vi "Main Tclk.vi"() -> ()   [LabVIEW 2018] (continued)
  T17 = cluster{"Filament (A)":sgl, "Accelerator Target (V)":sgl, "Accelerator Actual (V)":sgl, "Extrator Target (V)":sgl, "Extrator Actual (V)":sgl, "Emission Target (uA)":sgl, "Emission Actual (uA)":sgl, "Suppressor (V)":sgl, "Faraday I (nA)":sgl, "Lens1 Target (V)":sgl, "Lens1 Actual (V)":sgl, "Lens2 Target (V)":sgl, "Lens2 Actual (V)":sgl, "Gun Vac (Torr)":sgl, "Column Vac (Torr)":sgl, "Tip Lifetime (uAhr)":sgl}
  T18 = cluster{"Filament (A)":sgl, "Accelerator (V)":sgl, "AccI (uA)":sgl, "Extrator (V)":sgl, "Emission (uA)":sgl, "Suppressor (V)":sgl, "SuppI (uA)":sgl, "Lens1 (V)":sgl, "Lens1I (uA)":sgl, "Lens2 (V)":sgl, "Lens2I (uA)":sgl, "Tip Lifetime (hr)":sgl}
  T19 = cluster{"FIB mode":u8, "FIB focus":sgl, "FIB probe current":sgl, "FIB emission (uA)":sgl, "FIB rotation":sgl, "FIB aperture X":sgl, "FIB aperture Y":sgl, "FIB stig X":sgl, "FIB stig Y":sgl, "FIB beam shift X":sgl, "FIB beam shift Y":sgl}
  T20 = cluster{"Actual scan rate":dbl, "X resolution with rampdown":i32, "Actual sample rate":dbl, "Fetch backlog":dbl, "Total scan points":i32, "Frame rate (/s)":u32}
  T21 = cluster{"Reheat finish time":string, "Reheat Success":bool, "Initial emission (uA)":sgl, "Initial suppressor (V)":sgl, "V/I Slope":sgl}
  T22 = typedef "LVPoint32TypeDef.ctl" = cluster{"Horizontal":i32, "Vertical":i32}
  T23 = cluster{"FIB X coil":tag, "FIB Y coil":tag, "Beam blank":tag, "FIB Ext Scan":tag, "Detector":tag, "Shutter Drive":tag}
  T24 = enum32{"Hardware", "SEM", "Add'l SEM's", "File & Logging", "FIB Imaging", "FIB Reheat", "FIB Milling", "Alert"}
  T25 = cluster{"SEM X coil":refnum<k15>, "SEM Y coil":refnum<k15>, "FIB X coil":tag, "FIB Y coil":tag, "FIB Detector":tag, "SEM Detectors":refnum<k15>, "Det min (V)":dbl, "Det max (V)":dbl, "Eanable COM":bool, "COM port":refnum<visa-resource-name>, "FIB Beam blank":tag, "FIB Ext Scan":tag, "Det. FIB-NI auto switch":tag, "Shutter Drive":tag, "Machine Type":u8, "FIB Faraday Cup":tag, "Configuration file":path, "SEM Max FOV (um)":sgl, "Machine ID":string, "Save config file":bool, "Temperature port":refnum<visa-resource-name>, "Brightness A":dbl, "Contrast A":dbl, "Detector B name":string, "Brightness B":dbl, "Contrast B":dbl, "Logging Device":tag}
  T26 = cluster{"X size (um)":sgl, "Y size (um)":sgl, "X center (um)":sgl, "Y center (um)":sgl, "X size (V)":dbl, "X size auto":bool, "X stig":sgl[][], "Y stig":sgl[][], "X aln":sgl[][], "Y aln":sgl[][], "Scan rate (Hz)":u32, "Oversampling":u32, "Oversampling auto":bool, "Frame line rampdown ratio":sgl, "Pixel size (nm)":sgl, "WD (mm)":sgl[][], "X tiles":u8, "Y tiles":u8, "Overlap (um)":sgl, "Interlaced":bool, "dX (um)":sgl[], "dY (um)":sgl[], "Frames":u8}
  T27 = cluster{"GetInfo":bool, "Set Det A para":bool, "Set WD":bool, "Set Mag":bool, "Set stig":bool, "Set aln":bool, "Display":bool, "Save":bool, "8-bit":bool, "Detector A":bool, "Detector B":bool, "Detector C":bool, "Detector D":bool, "Inverse A":bool, "Inverse B":bool, "Inverse C":bool, "Inverse D":bool, "Inverse PNG":bool, "Freeze":bool, "PNG only":bool, "Upload":bool, "Delete after upload":bool}
  T28 = cluster{"Keep aspect ratio":bool, "Show Focus Index":bool, "Focus Index primary grid center":bool, "X Grids":u8[][], "Y Grids":u8[][], "Primary X index":u8[][], "Primary Y index":u8[][]}
  T29 = cluster{"Mid mag scan":bool, "Prior to main scan":bool, "Mid mag interval":u32, "X size (um)":sgl, "Y size (um)":sgl, "X center (um)":dbl, "Y center (um)":dbl, "Mid mag scan rate (Hz)":u32, "Pixel size (nm)":sgl, "Show MM box":bool}
  T30 = cluster{"Low mag scan":bool, "Prior to main scan":bool, "Low mag interval":u32, "Low mag scan FOV (micron)":dbl, "Low mag scan rate (Hz)":u32, "Show HM box":bool}
  T31 = cluster{"File path":path, "Notes":string, "Save recipe":bool, "Load recipe":bool, "Sample ID":string}
  T32 = cluster{"X resolution":u32, "Z resolution":u32, "X center":dbl, "Z center":dbl, "X size (V)":dbl, "Z size (V)":dbl, "Frame line rampdown ratio":dbl, "Scan rate (Hz)":u32, "Oversampling":u16}
  T33 = cluster{"Scan mode":u16, "Flip x":bool, "Flip z":bool, "Det":u16}
  T34 = cluster{"X resolution":u32, "Y resolution":u32, "X center":dbl, "Y center":dbl, "X size (V)":dbl, "Y size (V)":dbl, "Frame line rampdown ratio":dbl, "Scan rate (Hz)":u32, "Oversampling":u16}
  T35 = cluster{"X resolution":u32, "Z resolution":u32, "X offset (um)":sgl, "Z offset (um)":sgl, "X center (um)":sgl, "Z center (um)":sgl, "X size (um)":sgl, "Z size (um)":sgl, "UL-Ang":sgl, "UR-Ang":sgl, "Line milling time (s)":sgl, "Z-step (nm)":dbl, "Lines auto pause":u16, "Auto pause":bool, "Mill from Bottom":bool, "FIB FOV (um)":sgl, "Auto Profile":bool, "Mill start from Last":bool, "FIB PID on":bool, "FIB PID reset":bool, "FIB PID measured":u8, "FIB PID target":sgl, "FIB PID target slope":sgl, "FIB PID P":sgl, "FIB PID I":sgl, "FIB PID D":sgl, "Emission (uA)":dbl, "Suppressor (V)":sgl, "Auto reheat":bool}
  T36 = cluster{"3D imaging paused alarm":bool, "FIB emission warning":bool, "Low limit":dbl, "High limit":dbl, "Specimen @ SEM alarm":bool, "FIB CL current alarm":bool, "Beam Dump 1 alarm":bool, "Milling Z voltage alarm":bool, "EHT off alarm":bool, "Detector over scale warning":bool, "Image clipping alarm":bool, "Warning limit (um)":sgl, "Stop limit (um)":sgl, "Temperature alarm":bool, "Pause 3D-ING":bool, "Low limit (F)":sgl, "High limit (F)":sgl, "Temp limit auto":bool, "Delta (F)":sgl, "Gradient limit (F/min)":sgl, "SW error warning":bool, "Focus index warning":bool, "Focus index low limit":sgl, "Focus index stop limit":sgl, "Run Auto Stig":bool, "FI low limit auto":bool, "FI stop limit auto":bool}
  T37 = enum32{"All", "Detector A", "Detector B", "Detector A Low Mag", "Detector B Low Mag", "FIB", "FIB Milling Offset after Pause", "Auto Focus / Stig / Align", "Imaging Quality", "Temp. and Currents", "FIB HV Data", "Logging: Realtime Graphs"}
  T38 = cluster{cluster{"element":dbl, "A Img Focus Index":dbl}[]}[]
  T39 = cluster{"Log time array":u32[], "Delta X stop limit array":sgl[]}[]
  T40 = cluster{"Log time array":u32[], "Milling Y voltage array":sgl[]}
  T41 = cluster{"Log time array":u32[], "Delta Y stop limit array":sgl[]}[]
  T42 = cluster{sgl[][], sgl[][], sgl[][], sgl[][], sgl[][], sgl[], sgl[]}
  T43 = enum32{"Hardware", "SEM", "Add'l SEM's", "Data Logging", "FIB Imaging", "FIB Reheat", "FIB Milling", "Alert"}
  T44 = enum8{"Enabled", "Disabled", "Disabled and Grayed Out"}
  T45 = enum32{"Page Enabled", "Page Disabled", "Page Disabled & Grayed"}
  T46 = cluster{"Timestamp":timestamp, "Milling Z voltage":sgl, "FIB slice #":u32, "Pause for reheat":bool, "Last good FI":sgl, "Focus index":sgl, "SEM max FOV":sgl, "Remaining X shift frames":u32, "Remaining Y shift frames":u32}
  T47 = cluster{"left":i16, "top":i16, "right":i16, "bottom":i16}
  T48 = typedef "eventvkey.ctl" = enum16{"ASCII", "Enter", "Return", "Shift", "Ctrl", "Alt", "Cmd", "Opt", "Caps", "NumLock", "Clear", "Break", "Up", "Down", "Left", "Right", "Insert", "Delete", "Home", "End", "PageUp", "PageDown", "Escape", "Help", "Pause", "ScrollLock", "F1", "F2", "F3", "F4", "F5", "F6", "F7", "F8", "F9", "F10", "F11", "F12", "F13", "F14", "F15", "F16", "F17", "F18", "F19", "F20", "F21", "F22", "F23", "F24", "Play", "VolumeUp", "VolumeDown", "Mute", "Two Byte Char"}
  T49 = enum16{"open", "replace", "create", "open or create", "replace or create", "replace or create with confirmation"}
  T50 = enum16{"SEM", "FIB", "Mill", "SEM + FIB", "Mill + SEM", "Drift SEM", "Drift FIB", "None", "Ext", "Ext + SEM"}
  T51 = enum16{"Pages and Rows", "Pages and Columns", "Rows and Columns"}
  T52 = typedef "imagedata.ctl" = cluster{"image type":i32, "image depth":i32, "image":u8[], "mask":u8[], "colors":u32[], "Rectangle":cluster{"left":i16, "top":i16, "right":i16, "bottom":i16}}
  T53 = cluster{"A Img Focus Index":sgl[][], "B Img Focus Index":sgl[][], "C Img Focus Index":sgl[][], "D Img Focus Index":sgl[][]}
  T54 = cluster{"A Img Focus Index array":sgl[][][][], "B Img Focus Index array":sgl[][][][], "C Img Focus Index array":sgl[][][][], "D Img Focus Index array":sgl[][][][]}
  T55 = cluster{"SEM Status":cluster{"AO SampClk.MaxRate":dbl, "AI SampClk.MaxRate":dbl, "AO rate":dbl, "Scan speed":u8, "Detector #":u8, "X min (V)":dbl, "X max (V)":dbl, "X min index":i32, "X max index":i32, "AO multiline":u32, "Decimating factor":u16, "AvailSampPerChan":u32, "AO scan line":u32, "Total pixels recorded":i32, "Lines scanned":i32, "Scan time (m)":dbl, "Scan time (s)":dbl, "Remaining time (m)":u16, "Remaining time (s)":u8, "SEM Spec. I (nA)":sgl, "Frame":u8, "X tile":u8, "Y tile":u8}, "SEM Parameters":cluster{"Detector A":string, "Detector B":string, "Brightness A":sgl, "Contrast A":sgl, "Brightness B":sgl, "Contrast B":sgl, "Magnification":sgl, "Pixel size":sgl, "Working distance":sgl, "EHT":sgl, "Aperture":u8, "High current mode":u8, "Probe current":sgl, "Scan rotation":sgl, "Chamber vac":sgl, "Gun vac":sgl, "Beam shift X":sgl, "Beam shift Y":sgl, "Stig X":sgl, "Stig Y":sgl, "Alignment X":sgl, "Alignment Y":sgl, "Stage X":sgl, "Stage Y":sgl, "Stage Z":sgl, "Stage T":sgl, "Stage R":sgl, "Stage M":sgl}, "Image Focus Index":cluster{"A Img Focus Index":sgl, "B Img Focus Index":sgl, "C Img Focus Index":sgl, "D Img Focus Index":sgl}, "FIB parameters":cluster{"FIB mode":u8, "FIB focus":sgl, "FIB probe current":sgl, "FIB emission current":sgl, "FIB rotation":sgl, "FIB aperture X":sgl, "FIB aperture Y":sgl, "FIB stig X":sgl, "FIB stig Y":sgl, "FIB beam shift X":sgl, "FIB beam shift Y":sgl}, "Image Focus Index Array":cluster{"A Img Focus Index array":sgl[][], "B Img Focus Index array":sgl[][], "C Img Focus Index array":sgl[][], "D Img Focus Index array":sgl[][]}}
  T56 = cluster{"FIB mode":u8, "FIB focus":sgl, "FIB probe current":sgl, "FIB emission current":sgl, "FIB rotation":sgl, "FIB aperture X":sgl, "FIB aperture Y":sgl, "FIB stig X":sgl, "FIB stig Y":sgl, "FIB beam shift X":sgl, "FIB beam shift Y":sgl}
  T57 = cluster{u32[], "Faraday Cup high limit array":sgl[]}
  T58 = cluster{u32[], "Faraday Cup low limit array":sgl[]}
  T59 = cluster{u32[], "SEM Specimen I high limit array":sgl[]}
  T60 = cluster{u32[], "Specimen I high limit array":sgl[]}
  T61 = cluster{u32[], "Specimen I low limit array":sgl[]}
  T62 = cluster{u32[], "SEM Specimen I low limit array":sgl[]}
  T63 = cluster{u32[], "Milling I high limit array":sgl[]}
  T64 = cluster{u32[], "Milling I low limit array":sgl[]}
  T65 = cluster{u32[], "Faraday Cup low limit array":sgl[]}[]
  T66 = cluster{u32[], "Specimen I low limit array":sgl[]}[]
  T67 = cluster{u32[], "SEM Specimen I low limit array":sgl[]}[]
  T68 = cluster{u32[], "Milling I low limit array":sgl[]}[]
  T69 = typedef "LVRangeTypeDef.ctl" = cluster{"Minimum":dbl, "Maximum":dbl, "Increment":dbl, "Minor Increment":dbl, "Start":dbl}
  T70 = typedef "LVRectTypeDef.ctl" = cluster{"Left":i16, "Top":i16, "Right":i16, "Bottom":i16}
  T71 = cluster{u32[], "Delta X stop limit array":sgl[]}[]
  T72 = cluster{u32[], "Delta Y stop limit array":sgl[]}[]
  T73 = cluster{cluster{"Center":sgl, "A Img Focus Index":sgl}[]}
  T74 = cluster{cluster{"Center":sgl, "A Img Focus Index":sgl}[]}[]
  T75 = cluster{cluster{"Center":dbl, "A Img Focus Index":dbl}[]}[]
  T76 = cluster{"Timestamp":timestamp, "Last good milling Z voltage (V)":sgl, "FIB slice #":u32, "Pause for reheat":bool, "Last good FI":sgl, "Focus Index":sgl, "SEM Max FOV (um)":sgl, "Remaining X shift frames":u32, "Remaining Y shift frames":u32}
  T77 = cluster{"Shift":bool, "Ctrl":bool, "Alt":bool, "Cmd":bool, "Opt":bool}
  T78 = enum16{"Left Button", "Center Button", "Right Button", "Window Close"}
  T79 = cluster{"AI sampling time increment":dbl, "AI scaling coefficients":sgl[][], "AI channels":cluster{"AI 1":bool, "AI 2":bool, "AI 3":bool, "AI 4":bool}, "Resolution and scan":cluster{"X resolution":u32, "Z resolution":u32, "AI oversampling":u16, "Scan speed":u8, "Actual AO rate":dbl, "Frame line rampdown ratio":dbl, "X min (V)":dbl, "X max (V)":dbl, "Det min (V)":dbl, "Det max (V)":dbl}, "Decimating factor":u16, "Notes":string, "Other detectors":cluster{"Detector C name":string, "Detector D name":string}, "SEM parameters":cluster{"Detector A":string, "Detector B":string, "Brightness A":sgl, "Contrast A":sgl, "Brightness B":sgl, "Contrast B":sgl, "Magnification":sgl, "Pixel size":sgl, "Working distance":sgl, "EHT":sgl, "Aperture":u8, "High current mode":u8, "Probe current":sgl, "Scan rotation":sgl, "Chamber vac":sgl, "Gun vac":sgl, "Beam shift X":sgl, "Beam shift Y":sgl, "Stig X":sgl, "Stig Y":sgl, "Alignment X":sgl, "Alignment Y":sgl, "Stage X":sgl, "Stage Y":sgl, "Stage Z":sgl, "Stage T":sgl, "Stage R":sgl, "Stage M":sgl}, "FIB parameters":cluster{"FIB mode":u8, "FIB focus":sgl, "FIB probe current":u8, "FIB emission current":sgl, "FIB rotation":sgl, "FIB aperture X":sgl, "FIB aperture Y":sgl, "FIB stig X":sgl, "FIB stig Y":sgl, "FIB beam shift X":sgl, "FIB beam shift Y":sgl}, "Milling para":cluster{"X resolution":u32, "Z resolution":u32, "X offset (um)":sgl, "Z offset (um)":sgl, "X center (um)":sgl, "Z center (um)":sgl, "X size (um)":sgl, "Z size (um)":sgl, "UL-Ang":sgl, "UR-Ang":sgl, "Line milling time (s)":sgl, "Z-step (nm)":dbl, "Lines auto pause":u16, "Auto pause":bool, "Mill from Bottom":bool, "FIB FOV (um)":sgl, "Auto Profile":bool, "Mill start from Last":bool, "FIB PID on":bool, "FIB PID reset":bool, "FIB PID measured":u8, "FIB PID target":sgl, "FIB PID target slope":sgl, "FIB PID P":sgl, "FIB PID I":sgl, "FIB PID D":sgl, "Emission (uA)":dbl, "Suppressor (V)":sgl, "Auto reheat":bool}, "Machine ID":string, "Data Logging":cluster{"Temp (F)":sgl, "FIB Faraday Cup (nA)":sgl, "FIB Specimen I (nA)":sgl, "Beam Dump 1 (nA)":sgl, "Beam Dump 2 (nA)":sgl, "Milling I (nA)":sgl, "SEM Specimen I (nA)":sgl, "Milling Z voltage (V)":sgl, "Focus Index":sgl, "FIB slice #":u32}}
  T80 = cluster{"FIB mode":u8, "FIB focus":sgl, "FIB probe current":u8, "FIB emission current":sgl, "FIB rotation":sgl, "FIB aperture X":sgl, "FIB aperture Y":sgl, "FIB stig X":sgl, "FIB stig Y":sgl, "FIB beam shift X":sgl, "FIB beam shift Y":sgl}
  T81 = cluster{"Temp (F)":sgl, "FIB Faraday Cup (nA)":sgl, "FIB Specimen I (nA)":sgl, "Beam Dump 1 (nA)":sgl, "Beam Dump 2 (nA)":sgl, "Milling I (nA)":sgl, "SEM Specimen I (nA)":sgl, "Milling Z voltage (V)":sgl, "Focus Index":sgl, "FIB slice #":u32}
  T82 = typedef "DialogType.ctl" = u16
  T83 = cluster{"Log time array":u32[], "Focus index array":sgl[]}
  T84 = cluster{"Log time array":u32[], "FI low limit array":sgl[]}
  T85 = cluster{"Log time array":u32[], "FI low limit array":sgl[]}[]
  T86 = cluster{"Log time array":u32[], "FRC array":sgl[]}
  T87 = cluster{"Log time array":u32[], "FRC array":sgl[]}[]
  T88 = cluster{"Log time array":u32[], "Delta X array":sgl[]}
  T89 = cluster{"Log time array":u32[], "Delta X stop limit array":sgl[]}
  T90 = cluster{"Log time array":u32[], "Delta X sum array":sgl[]}
  T91 = cluster{"Log time array":u32[], "Delta X sum array":sgl[]}[]
  T92 = cluster{"Log time array":u32[], "Delta Y array":sgl[]}
  T93 = cluster{"Log time array":u32[], "Delta Y sum array":sgl[]}
  T94 = cluster{"Log time array":u32[], "Delta Y sum array":sgl[]}[]
  T95 = cluster{"Log time array":u32[], "Delta Z array":sgl[]}
  T96 = cluster{"Log time array":u32[], "Milling Z voltage array":sgl[]}
  T97 = cluster{"Log time array":u32[], "Delta image array":sgl[]}
  T98 = cluster{"Log time array":u32[], "Specimen I array":sgl[]}
  T99 = cluster{"Log time array":u32[], "Specimen I high limit array":sgl[]}
  T100 = cluster{"Log time array":u32[], "Specimen I low limit array":sgl[]}
  T101 = cluster{"Log time array":u32[], "Specimen I low limit array":sgl[]}[]
  T102 = cluster{"Log time array":u32[], "SEM Specimen I array":sgl[]}
  T103 = cluster{"Log time array":u32[], "SEM Specimen I high limit array":sgl[]}
  T104 = cluster{"Log time array":u32[], "SEM Specimen I low limit array":sgl[]}
  T105 = cluster{"Log time array":u32[], "SEM Specimen I low limit array":sgl[]}[]
  T106 = cluster{"Log time array":u32[], "Beam Dump 2 array":sgl[]}
  T107 = cluster{"Log time array":u32[], "BD2 high limit array":sgl[]}
  T108 = cluster{"Log time array":u32[], "BD2 low limit array":sgl[]}
  T109 = cluster{"Log time array":u32[], "BD2 low limit array":sgl[]}[]
  T110 = cluster{"Log time array":u32[], "Milling I array":sgl[]}
  T111 = cluster{"Log time array":u32[], "Milling I high limit array":sgl[]}
  T112 = cluster{"Log time array":u32[], "Milling I low limit array":sgl[]}
  T113 = cluster{"Log time array":u32[], "Milling I low limit array":sgl[]}[]
  T114 = cluster{"Log time array":u32[], "Beam Dump 1 array":sgl[]}
  T115 = cluster{"Log time array":u32[], "BD1 high limit array":sgl[]}
  T116 = cluster{"Log time array":u32[], "BD1 low limit array":sgl[]}
  T117 = cluster{"Log time array":u32[], "BD1 low limit array":sgl[]}[]
  T118 = cluster{"Filament (A)":sgl, "Acclerator (V)":sgl, "AccI (uA)":sgl, "Extractor (V)":sgl, "Emission (uA)":sgl, "Suppressor (V)":sgl, "SuppI (uA)":sgl, "Lens1 (V)":sgl, "Lens1I (uA)":sgl, "Lens2 (V)":sgl, "Lens2I (uA)":sgl, "Tip Lifetime (hr)":sgl}
  T119 = cluster{"SEM Scan Parameters":cluster{"X size (um)":sgl, "Y size (um)":sgl, "X center (um)":dbl, "Y center (um)":dbl, "X size (V)":dbl, "X size auto":bool, "X stig":sgl[][], "Y stig":sgl[][], "X aln":sgl[][], "Y aln":sgl[][], "Scan rate (Hz)":u32, "Oversampling":u32, "Oversampling auto":bool, "Frame line rampdown ratio":sgl, "Pixel size (nm)":sgl, "WD (mm)":sgl[][], "X tiles":u8, "Y tiles":u8, "Overlap (um)":sgl, "Interlaced":bool, "dX (um)":sgl[], "dY (um)":sgl[], "Frames":u8}, "Detector Information":cluster{"Brightness A":dbl, "Contrast A":dbl, "Detector B name":string, "Brightness B":dbl, "Contrast B":dbl, "Detector C name":string, "Detector D name":string}, "SEM Options":cluster{"GetInfo":bool, "Set Det A para":bool, "Set WD":bool, "Set Mag":bool, "Set stig":bool, "Set aln":bool, "Display":bool, "Save":bool, "8-bit":bool, "Detector A":bool, "Detector B":bool, "Detector C":bool, "Detector D":bool, "Inverse A":bool, "Inverse B":bool, "Inverse C":bool, "Inverse D":bool, "Inverse PNG":bool, "Freeze":bool, "PNG only":bool, "Upload":bool, "Delete after upload":bool}, "Focus Index Options":cluster{"Keep aspect ratio":bool, "Show Focus Index":bool, "Focus Index primary grid center":bool, "X Grids":u8[][], "Y Grids":u8[][], "Primary X index":u8[][], "Primary Y index":u8[][]}, "Image fit to":u8, "File Information":cluster{"File path":path, "Notes":string, "Save recipe":bool, "Load recipe":bool, "Sample ID":string}, "Low mag SEM":cluster{"Low mag scan":bool, "Prior to main scan":bool, "Low mag interval":u32, "Low mag scan FOV (micron)":dbl, "Low mag scan rate (Hz)":u32, "Show HM box":bool}, "Mid Mag SEM":cluster{"Mid mag scan":bool, "Prior to main scan":bool, "Mid mag interval":u32, "X size (um)":sgl, "Y size (um)":sgl, "X center (um)":dbl, "Y center (um)":dbl, "Mid mag scan rate (Hz)":u32, "Pixel size (nm)":dbl, "Show MM box":bool}, "FIB-SEM Angle":dbl, "Milling para":cluster{"X resolution":u32, "Z resolution":u32, "X offset (um)":sgl, "Z offset (um)":sgl, "X center (um)":sgl, "Z center (um)":sgl, "X size (um)":sgl, "Z size (um)":sgl, "UL-Ang":sgl, "UR-Ang":sgl, "Line milling time (s)":sgl, "Z-step (nm)":dbl, "Lines auto pause":u16, "Auto pause":bool, "Mill from Bottom":bool, "FIB FOV (um)":sgl, "Auto Profile":bool, "Mill start from Last":bool, "FIB PID on":bool, "FIB PID reset":bool, "FIB PID measured":u8, "FIB PID target":sgl, "FIB PID target slope":sgl, "FIB PID P":sgl, "FIB PID I":sgl, "FIB PID D":sgl, "Emission (uA)":dbl, "Suppressor (V)":sgl, "Auto reheat":bool}, "FI Detector":u16, "Auto Optimzation":bool, "Images per Auto Optimization":u16, "AF Range (nm)":sgl, "AF Steps":u8, "AS Range (%)":sgl, "AS Steps":u8, "AA Range (%)":sgl, "AA Steps":u8, "X shift (nm/frame)":dbl, "Y shift (nm/frame)":dbl, "FIB Y zoom pixel (nm)":dbl, "Mail server":string, "Email Alert Recipients":string[], "Alert Settings":cluster{"3D imaging paused alarm":bool, "FIB emission limit warning":bool, "Low limit":sgl, "High limit":sgl, "Specimen @ SEM alarm":bool, "FIB CL current alarm":bool, "Beam Dump 1 alarm":bool, "Milling Z voltage alarm":bool, "EHT off alarm":bool, "Detector over scale warning":bool, "Image clipping alarm":bool, "Warning limit (um)":sgl, "Stop limit (um)":sgl, "Temperature alarm":bool, "Pause 3D-ING":bool, "Low limit (F)":sgl, "High limit (F)":sgl, "Temp limit auto":bool, "Delta (F)":sgl, "Gradient limit (F/min)":sgl, "SW error warning":bool, "Focus index warning":bool, "Focus index low limit":sgl, "Focus index stop limit":sgl, "Run Auto Stig":bool, "FI low limit auto":bool, "FI stop limit auto":bool}, "Reheat Parameters":cluster{"Filament I (A)":sgl, "Reheat time (s)":sgl, "Emission (uA)":sgl, "Calculate V/I slope":bool, "Pre-calc delay (min)":sgl, "Disable Reheat Retries":bool, "Restore Voltages":bool}, "Start FIB HV DataLog":bool, "Interval (s)":u16}
  T120 = cluster{"Mid mag scan":bool, "Prior to main scan":bool, "Mid mag interval":u32, "X size (um)":sgl, "Y size (um)":sgl, "X center (um)":dbl, "Y center (um)":dbl, "Mid mag scan rate (Hz)":u32, "Pixel size (nm)":dbl, "Show MM box":bool}
  T121 = cluster{"3D imaging paused alarm":bool, "FIB emission limit warning":bool, "Low limit":sgl, "High limit":sgl, "Specimen @ SEM alarm":bool, "FIB CL current alarm":bool, "Beam Dump 1 alarm":bool, "Milling Z voltage alarm":bool, "EHT off alarm":bool, "Detector over scale warning":bool, "Image clipping alarm":bool, "Warning limit (um)":sgl, "Stop limit (um)":sgl, "Temperature alarm":bool, "Pause 3D-ING":bool, "Low limit (F)":sgl, "High limit (F)":sgl, "Temp limit auto":bool, "Delta (F)":sgl, "Gradient limit (F/min)":sgl, "SW error warning":bool, "Focus index warning":bool, "Focus index low limit":sgl, "Focus index stop limit":sgl, "Run Auto Stig":bool, "FI low limit auto":bool, "FI stop limit auto":bool}
  T122 = cluster{"Suppressor (V)":sgl, "Emission (uA)":sgl}
  T123 = cluster{"Suppressor (V)":sgl, "Emission Actual (uA)":sgl}
diagram:
  n1 = stacked-sequence {
    frame #0 {
      n2 = disable-structure shown="Disabled" {
        frame Disabled {
          w17 = string[] ["Machine ID", "Machine type", "SEM maximum FOV (um)", "Detector min (V)", "Detector max (V)", "Brightness A", "Contrast A", "Detector B name", "Brightness B", "Contrast B"]
          n3 = local read "Hardware Configuration"() -> (w85:T25)
          n4 = Unbundle By Name(w85) -> ("Configuration file"=w86:path)
          n5 = call-poly <vilib>:"Read From Spreadsheet File.vi"("delimiter (\\t)"="," ("delimiter (\\t)"), "file path (dialog if empty)"=w86) -> ("all rows"=w18:string[][])  [unwired: 5 in, 4 out]
          n6 = Index Array(array=w17, index=0) -> (element=w43:string)
          n7 = Index Array(array=w17, index=1) -> (element=w40:string)
          n8 = Index Array(array=w17, index=2) -> (element=w31:string)
          n9 = Index Array(array=w17, index=3) -> (element=w29:string)
          n10 = Index Array(array=w17, index=4) -> (element=w30:string)
          n11 = Index Array(array=w17, index=5) -> (element=w28:string)
          n12 = Index Array(array=w17, index=6) -> (element=w27:string)
          n13 = Index Array(array=w17, index=7) -> (element=w26:string)
          n14 = Index Array(array=w17, index=8) -> (element=w25:string)
          n15 = Index Array(array=w17, index=9) -> (element=w24:string)
          n16 = call "2D array search.vi"("Search For"=w43, "Input Array"=w18) -> ("Column"=w56:i32, "Row"=w55:i32)  [unwired: 7 in, 1 out]
          n17 = call "2D array search.vi"("Search For"=w40, "Input Array"=w18) -> ("Column"=w77:i32, "Row"=w78:i32)  [unwired: 7 in, 1 out]
          n18 = call "2D array search.vi"("Search For"=w31, "Input Array"=w18) -> ("Column"=w75:i32, "Row"=w74:i32)  [unwired: 7 in, 1 out]
          n19 = call "2D array search.vi"("Search For"=w29, "Input Array"=w18) -> ("Column"=w48:i32, "Row"=w50:i32)  [unwired: 7 in, 1 out]
          n20 = call "2D array search.vi"("Search For"=w30, "Input Array"=w18) -> ("Column"=w51:i32, "Row"=w53:i32)  [unwired: 7 in, 1 out]
          n21 = call "2D array search.vi"("Search For"=w28, "Input Array"=w18) -> ("Column"=w72:i32, "Row"=w70:i32)  [unwired: 7 in, 1 out]
          n22 = call "2D array search.vi"("Search For"=w27, "Input Array"=w18) -> ("Column"=w69:i32, "Row"=w67:i32)  [unwired: 7 in, 1 out]
          n23 = call "2D array search.vi"("Search For"=w26, "Input Array"=w18) -> ("Column"=w66:i32, "Row"=w64:i32)  [unwired: 7 in, 1 out]
          n24 = call "2D array search.vi"("Search For"=w25, "Input Array"=w18) -> ("Column"=w63:i32, "Row"=w61:i32)  [unwired: 7 in, 1 out]
          n25 = call "2D array search.vi"("Search For"=w24, "Input Array"=w18) -> ("Column"=w60:i32, "Row"=w58:i32)  [unwired: 7 in, 1 out]
          n26 = Increment(x=w56) -> (x+1=w57:i32)
          n27 = Increment(x=w77) -> (x+1=w76:i32)
          n28 = Increment(x=w75) -> (x+1=w73:i32)
          n29 = Increment(x=w48) -> (x+1=w49:i32)
          n30 = Increment(x=w51) -> (x+1=w52:i32)
          n31 = Increment(x=w72) -> (x+1=w71:i32)
          n32 = Increment(x=w69) -> (x+1=w68:i32)
          n33 = Increment(x=w66) -> (x+1=w65:i32)
          n34 = Increment(x=w63) -> (x+1=w62:i32)
          n35 = Increment(x=w60) -> (x+1=w59:i32)
          n36 = Index Array(array=w18, index (row)=w55, index (col)=w57) -> (element=w54:string)
          n37 = Index Array(array=w18, index (row)=w78, index (col)=w76) -> (element=w88:string)
          n38 = Index Array(array=w18, index (row)=w74, index (col)=w73) -> (element=w80:string)
          n39 = Index Array(array=w18, index (row)=w50, index (col)=w49) -> (element=w47:string)
          n40 = Index Array(array=w18, index (row)=w53, index (col)=w52) -> (element=w46:string)
          n41 = Index Array(array=w18, index (row)=w70, index (col)=w71) -> (element=w84:string)
          n42 = Index Array(array=w18, index (row)=w67, index (col)=w68) -> (element=w83:string)
          n43 = Index Array(array=w18, index (row)=w64, index (col)=w65) -> (element=w21:string)
          n44 = Index Array(array=w18, index (row)=w61, index (col)=w62) -> (element=w81:string)
          n45 = Index Array(array=w18, index (row)=w58, index (col)=w59) -> (element=w82:string)
          n46 = case shown="\"Feiss\", Default" w88 {
            tunnel: [u8 0 ("Machine Type") u8 2 ("Machine Type") u8 1 ("Machine Type")] -> w87
            frame "Feiss", Default {
            }
            frame "Jeiss" {
            }
            frame "NVision" {
            }
          }
          n47 = Fract/Exp String To Number(string=w80) -> (number=w79:dbl)  [unwired: 4 out]
          n48 = Fract/Exp String To Number(string=w47) -> (number=w45:dbl)  [unwired: 4 out]
          n49 = Fract/Exp String To Number(string=w46) -> (number=w44:dbl)  [unwired: 4 out]
          n50 = Fract/Exp String To Number(string=w84) -> (number=w23:dbl)  [unwired: 4 out]
          n51 = Fract/Exp String To Number(string=w83) -> (number=w22:dbl)  [unwired: 4 out]
          n52 = Fract/Exp String To Number(string=w81) -> (number=w20:dbl)  [unwired: 4 out]
          n53 = Fract/Exp String To Number(string=w82) -> (number=w19:dbl)  [unwired: 4 out]
          n54 = Bundle By Name(cluster=w85, "Machine ID"=w54, "Machine Type"=w87, "SEM Max FOV (um)"=w79, "Det min (V)"=w45, "Det max (V)"=w44, "Brightness A"=w23, "Contrast A"=w22, "Detector B name"=w21, "Brightness B"=w20, "Contrast B"=w19) -> (w89:T25)
          n55 = local write "Hardware Configuration"(w89) -> ()
          "HW config items" <- w17
        }
        frame Enabled {
        }
      }
      n56 = flat-sequence {
        frame #0 {
          n57 = local read "Hardware Configuration"() -> (w2:T25)
          n58 = shared-variable ".\\Zeiss Library.lvlib\\SW date"("SW date") -> ()  [unwired: 1 in, 1 out]
          n59 = call "Read Config Settings from INI file.vi"("Hardware Configuration"=w2) -> ("Hardware Configuration Out"=w3:T25)  [unwired: 9 in]
          n60 = local write "Hardware Configuration"(w3) -> ()
        }
        frame #1 {
          n61 = local read "SEM HW Config"() -> (w4:T9)
          n62 = local read "FIB HW Config"() -> (w12:T23)
          n63 = Unbundle By Name(w4) -> ("SEM X coil"=w5:refnum<k15>)
          n64 = Unbundle By Name(w12) -> ("FIB X coil"=w13:tag)
          n65 = Type Cast(x=w5) -> (*(type *) &x=w6:string)  [unwired: 1 in]
          n66 = Type Cast(x=w13) -> (*(type *) &x=w11:string)  [unwired: 1 in]
          n67 = Match Pattern(string=w6, regular expression="/") -> (before substring=w8:string)  [unwired: 1 in, 3 out]
          n68 = Match Pattern(string=w11, regular expression="/") -> (before substring=w9:string)  [unwired: 1 in, 3 out]
          n69 = call <vilib>:"DAQmx Reset Device.vi"("device in"=w8) -> ()  [unwired: 14 in, 1 out]
          n70 = call <vilib>:"DAQmx Reset Device.vi"("device in"=w9) -> ()  [unwired: 14 in, 1 out]
        }
        frame #2 {
          w14 = u16 1 items=["Do Nothing", "Send Idle Only", "Watch FIB & SEM", "Watch FIB Only", "Watch SEM Only"] ("WatchDog Mode")
          n71 = shared-variable ".\\Zeiss Library.lvlib\\Force tclk init"(TRUE ("Force tclk init")) -> ()  [unwired: 1 in, 1 out]
          n72 = call "FM Gen Pulse for FIB-SEM.vi"("WatchDog Mode"=w14, "State Value"=i16 0) -> ()  [unwired: 7 in, 3 out]
        }
      }
    }
    frame #1 {
      w174 = sgl[][] [] ("FI array")
      w96 = bool[][] [[FALSE]] ("AF Success tiled")
      w222 = FALSE ("Visible")
      w113 = path "D:/3D FIB-SEM Files" ("path")
      w172 = sgl[][][] [] ("FI grid array")
      w132 = u32[] [] ("FI array")
      w105 = sgl 20.0 ("t")
      w199 = T44."Disabled and Grayed Out" ("Disabled")
      w110 = FALSE ("Save recipe")
      w95 = sgl[] [] ("FI array")
      w111 = TRUE ("Auto Optimzation")
      w103 = T44."Enabled" ("Disabled")
      w240 = FALSE ("Auto pause")
      w97 = u32 0 ("FIB slice #")
      w99 = FALSE ("Off")
      n73 = local write "Delta Z array"(w95) -> ()
      n74 = local write "Delta X sum array"(w95) -> ()
      n75 = local write "Delta Y sum array"(w95) -> ()
      n76 = local write "Delta image array"(w95) -> ()
      n77 = local write "Milling Z voltage array"(w95) -> ()
      n78 = local write "Re-engage Delta X array"(w95) -> ()
      n79 = local write "Re-engage Delta Y array"(w95) -> ()
      n80 = local write "Re-engage X shift array"(w95) -> ()
      n81 = local write "Re-engage Y shift array"(w95) -> ()
      n82 = local write "Temp array"(w95) -> ()
      n83 = local write "Faraday Cup array"(w95) -> ()
      n84 = local write "SEM Specimen I array"(w95) -> ()
      n85 = local write "Beam Dump 1 array"(w95) -> ()
      n86 = local write "Beam Dump 2 array"(w95) -> ()
      n87 = local write "Milling I array"(w95) -> ()
      n88 = local write "Focus index array"(w95) -> ()
      n89 = local write "FRC array"(w95) -> ()
      n90 = local write "Delta X array"(w95) -> ()
      n91 = local write "Delta Y array"(w95) -> ()
      n92 = local write "Specimen I array"(w95) -> ()
      n93 = To Variant(anything=T20 {"Actual scan rate"=0.0, "X resolution with rampdown"=0, "Actual sample rate"=0.0, "Fetch backlog"=0.0, "Total scan points"=0, "Frame rate (/s)"=0} ("type")) -> (Variant=w318:variant)
      n94 = local read "SEM Status"() -> (w307:T12)
      n95 = shared-variable ".\\Zeiss Library.lvlib\\Realtime Imaging Info"(w318) -> ()  [unwired: 1 in, 1 out]
      n96 = To Variant(anything=w307) -> (Variant=w306:variant)
      n97 = Unbundle By Name("Hardware Configuration") -> ("SEM X coil"=w263:refnum<k15>, "SEM Y coil"=w312:refnum<k15>, "FIB X coil"=w313:tag, "FIB Y coil"=w314:tag, "FIB Detector"=w315:tag, "SEM Detectors"=w261:refnum<k15>, "Det min (V)"=w309:dbl, "Det max (V)"=w310:dbl, "Eanable COM"=w256:bool, "COM port"=w311:refnum<visa-resource-name>, "FIB Beam blank"=w299:tag, "FIB Ext Scan"=w296:tag, "Det. FIB-NI auto switch"=w300:tag, "Shutter Drive"=w100:tag, "Machine Type"=w289:u8, "Machine ID"=w165:string, "Logging Device"=w248:tag)
      "COM port" <- w311
      "Machine Type" <- w289
      "Log Device" <- w248
      "Shutter Drive Local?" <- w100
      n98 = shared-variable ".\\Zeiss Library.lvlib\\SEMInfo"(w306) -> ()  [unwired: 2 out]
      n99 = local write "Temp high limit array"(w95) -> ()
      n100 = local write "Temp low limit array"(w95) -> ()
      n101 = local write "Specimen I high limit array"(w95) -> ()
      n102 = local write "Specimen I low limit array"(w95) -> ()
      n103 = local write "SEM Specimen I high limit array"(w95) -> ()
      n104 = local write "SEM Specimen I low limit array"(w95) -> ()
      n105 = local write "FI low limit array"(w95) -> ()
      n106 = local write "Faraday Cup high limit array"(w95) -> ()
      n107 = local write "Faraday Cup low limit array"(w95) -> ()
      n108 = local write "Image Tabs"(T37."All" ("Image Tabs")) -> ()
      n109 = local write "Stig Options"(enum16{"Defaut", "Stig X", "Stig Y"}."Defaut" ("Stig Options")) -> ()
      n110 = local write "Log time array"(w132) -> ()
      n111 = local write "Cycle time array"(w132) -> ()
      n112 = local write "Cycle time est offset array"(i16[] [] ("FI array")) -> ()
      n113 = call <instrlib>:"niFgen Initialize.vi"("Resource Name"=w263) -> ("error out"=w264:errorcluster, "Instrument Handle Out"=w274:refnum<k15>)  [unwired: 9 in]
      n114 = call <instrlib>:"niScope Initialize.vi"("resource name"=w261) -> ("instrument handle"=w275:refnum<k15>, "error out"=w270:errorcluster)  [unwired: 13 in]
      n115 = case shown="2" w289 {
        tunnel: [10.0 ("X size (V)") 20.0 ("X size (V)") 16.0 ("X size (V)")] -> w293
        tunnel: [90.0 ("X size (V)") 54.0 ("X size (V)") 90.0 ("X size (V)")] -> w292
        tunnel: [500.0 ("X size (V)") 382.193 ("FIB FOV (um)") 500.0 ("X size (V)")] -> w258
        tunnel: [w583 w599 w624] -> w282
        tunnel: [w585 w599 w624] -> w281
        tunnel: [w585 w599 w617] -> w181
        tunnel: ["Low limit (uA)" ("Label.Text") "Low limit (uA)" ("Label.Text") "Low limit (uA)" ("Label.Text")] -> w224
        tunnel: ["High limit (uA)" ("Label.Text") "High limit (uA)" ("Label.Text") "High limit (uA)" ("Label.Text")] -> w223
        tunnel: ["Faraday" ("Label.Text") " B.D. -\n Spec." ("Label.Text") "Faraday" ("Label.Text")] -> w221
        tunnel: ["Faraday Cup (nA)" ("Label.Text") "B.D. - Spec. (nA)" ("Label.Text") "Faraday Cup (nA)" ("Label.Text")] -> w220
        tunnel: [1.4 ("X size (V)") 1.2 ("X size (V)") 1.38 ("X size (V)")] -> w214
        tunnel: [2.0 ("X size (V)") 1.8 ("X size (V)") 2.0 ("X size (V)")] -> w213
        tunnel: [w583 w597 w624] -> w188
        tunnel: [T45."Page Enabled" ("Page Enabled State") T45."Page Disabled & Grayed" ("Page Enabled State") T45."Page Enabled" ("Page Enabled State")] -> w127
        tunnel: [w585 w599 w624] -> w160
        tunnel: [w583 w597 w617] -> w159
        tunnel: [w585 w597 w624] -> w101
        tunnel: [w583 w597 w617] -> w158
        tunnel: [w585 w597 w617] -> w151
        tunnel: [sgl 6.0 ("Overhead (s)") sgl 7.0 ("Overhead (s)") sgl 5.0 ("Overhead (s)")] -> w150
        frame 0, Default {
          w586 = T44."Enabled" ("Disabled")
          w583 = TRUE ("data")
          w585 = FALSE ("data")
          # "Feiss"
          n116 = property on="Turn on FIB gun" class="Bool (strict)"("DisabledEnum"=w586) -> ()  [unwired: 2 in, 2 out]
          n117 = property on="Request to reheat" class="Bool (strict)"("DisabledEnum"=w586) -> ()  [unwired: 2 in, 2 out]
        }
        frame 1 {
          w597 = FALSE ("data")
          w599 = TRUE ("data")
          # "NVision"
        }
        frame 2 {
          w624 = TRUE ("data")
          w617 = FALSE ("data")
          # "Jeiss"
          n118 = invoke class="_EMApi" method="InitialiseRemoting"(reference="Api") -> (reference out=w648:refnum<k7>, error out=w647:errorcluster, "InitialiseRemoting"=w660:i32)  [unwired: 2 in]
          n119 = call "SmartSEM Remote API set float.vi"("error in"=w647, "vValue"=sgl 0.0, "lpszParam"="DP_FIB_LOCK_MAG", "ActiveX Container"=w648) -> ("error out"=w643:errorcluster, "reference out"=w644:refnum<k7>)  [unwired: 6 in]
          n120 = call "SmartSEM Remote API set string.vi"("error in"=w643, "vValue"="Polaroid 545" ("lpszParam"), "lpszParam"="DP_USE_REF_MAG", "ActiveX Container"=w644) -> ("error out"=w639:errorcluster, "reference out"=w640:refnum<k7>)  [unwired: 6 in]
          n121 = Equal To 0?(x=w660) -> (x = 0?=w659:bool)
          n122 = case shown="True" w659 {
            frame False {
            }
            frame True {
              n123 = local write "Status message"("API Initialized" ("Status message")) -> ()
            }
          }
          n124 = call "SmartSEM Remote API set string.vi"("error in"=w639, "vValue"="Undefined" ("lpszParam"), "lpszParam"="DP_FIB_MILL_PROBE", "ActiveX Container"=w640) -> ("error out"=w628:errorcluster, "reference out"=w627:refnum<k7>)  [unwired: 6 in]
          n125 = call "SmartSEM Remote API get string.vi"("error in"=w628, "lpszParam"="DP_FIB_IMAGE_PROBE", "ActiveX Container"=w627) -> ("error out"=w622:errorcluster, "data"=w635:string, "reference out"=w623:refnum<k7>)  [unwired: 6 in]
          n126 = local write "FIB Milling Probe"(w635) -> ()
          n127 = call "SmartSEM Remote API get float.vi"("error in"=w622, "lpszParam"="AP_FIB_OBJECTIVE_POTENTIAL", "ActiveX Container"=w623) -> ("error out"=w620:errorcluster, "vValue"=w618:sgl, "reference out"=w621:refnum<k7>)  [unwired: 6 in]
          n128 = call "SmartSEM Remote API set float.vi"("error in"=w620, "vValue"=sgl 1.0, "lpszParam"="DP_AUTO_HYSTERESIS", "ActiveX Container"=w621) -> ("error out"=w613:errorcluster, "reference out"=w612:refnum<k7>)  [unwired: 6 in]
          n129 = call "SmartSEM Remote API set float.vi"("error in"=w613, "vValue"=sgl 1.0, "lpszParam"="DP_POINT_USING", "ActiveX Container"=w612) -> ("error out"=w610:errorcluster, "reference out"=w611:refnum<k7>)  [unwired: 6 in]
          n130 = call "SmartSEM Remote API set float.vi"("error in"=w610, "vValue"=sgl 0.0, "lpszParam"="DP_PANEL_DISABLE", "ActiveX Container"=w611) -> ("error out"=w630:errorcluster, "reference out"=w653:refnum<k7>)  [unwired: 6 in]
          n131 = call "SmartSEM Remote API set float.vi"("error in"=w630, "vValue"=sgl 0.0, "lpszParam"="DP_JOYSTICK_DISABLE", "ActiveX Container"=w653) -> ("error out"=w629:errorcluster, "reference out"=w633:refnum<k7>)  [unwired: 6 in]
          n132 = call "SmartSEM Remote API get string.vi"("error in"=w629, "lpszParam"="SV_VERSION", "ActiveX Container"=w633) -> ("data"=w634:string, "reference out"=w631:refnum<k7>)  [unwired: 6 in, 1 out]
          n133 = Scan From String(format string="V%f", input string=w634) -> (output 1=w651:dbl)  [unwired: 3 in, 3 out]
          n134 = Greater Or Equal?(x=w651, y=6.01) -> (x >= y?=w649:bool)
          n135 = case shown="True" w649 {
            tunnel: w631 -> [_ w671]
            frame False {
            }
            frame True {
              n136 = call "SmartSEM Remote API set float.vi"("vValue"=sgl 1.0, "lpszParam"="DP_FIB_SCAN_ROT", "ActiveX Container"=w671) -> ()  [unwired: 7 in, 2 out]
            }
          }
          n137 = local write "FIB Milling Objective (V)"(w618) -> ()
        }
      }
      "Overhead (s)" <- w150
      n138 = local write "BD1 high limit array"(w95) -> ()
      n139 = local write "BD1 low limit array"(w95) -> ()
      n140 = local write "BD2 high limit array"(w95) -> ()
      n141 = local write "BD2 low limit array"(w95) -> ()
      n142 = local write "Milling I high limit array"(w95) -> ()
      n143 = local write "Milling I low limit array"(w95) -> ()
      n144 = property class="niScope"(reference=w275, error in=w270) -> (reference out=w271:refnum<k15>, error out=w269:errorcluster, "Maximum Real Time Sample Rate"=w260:dbl)
      n145 = property class="niFgen"(reference=w274, error in=w264) -> (reference out=w266:refnum<k15>, error out=w265:errorcluster, "Sample Rate"=w262:dbl)
      n146 = Bundle By Name(cluster="SEM HW Config", "SEM X coil"=w263, "SEM Y coil"=w312, "Detectors A&B"=w261, "Det min (V)"=w309, "Det max (V)"=w310, "Eanable COM"=w256, "COM port"=w311, "Detector FIB-NI auto switch"=w300, "Machine Type"=w289, "Machine ID"=w165) -> (w276:T9)
      n147 = call "FIB ext scan.vi"("Ext on"=FALSE ("data"), "FIB Ext Scan"=w296) -> ()  [unwired: 9 in, 1 out]
      n148 = call <instrlib>:"niFgen Abort Generation.vi"("error in (no error)"=w265, "Instrument Handle"=w266) -> ("error out"=w268:errorcluster, "Instrument Handle Out"=w267:refnum<k15>)  [unwired: 8 in]
      n149 = call <instrlib>:"niFgen Close.vi"("error in (no error)"=w268, "Instrument Handle"=w267) -> ()  [unwired: 9 in, 1 out]
      n150 = Bundle By Name(cluster="FIB HW Config", "FIB X coil"=w313, "FIB Y coil"=w314, "Beam blank"=w299, "FIB Ext Scan"=w296, "Detector"=w315, "Shutter Drive"=w100) -> (w317:T23)
      n151 = local read "Api"() -> (w109:refnum<k7>)
      n152 = call <instrlib>:"niScope Abort.vi"("instrument handle"=w271, "error in"=w269) -> ("instrument handle out"=w273:refnum<k15>, "error out"=w272:errorcluster)  [unwired: 12 in]
      n153 = call "FIB beam blank.vi"("ActiveX Container"=w109, "Beam blanked"=TRUE, "lines"=w299) -> ()  [unwired: 2 in, 1 out]
      n154 = call <instrlib>:"niScope Close.vi"("instrument handle"=w273, "error in"=w272) -> ()  [unwired: 13 in, 1 out]
      n155 = local write "SEM HW Config"(w276) -> ()
      n156 = local read "SEM Status"() -> (w303:T12)
      n157 = Bundle By Name(cluster=w303, "AO SampClk.MaxRate"=w262, "AI SampClk.MaxRate"=w260) -> (w304:T12)
      n158 = case shown="False" w256 {
        tunnel: [T44."Disabled and Grayed Out" ("Disabled") T44."Enabled" ("Disabled")] -> w257
        frame False {
        }
        frame True {
        }
      }
      n159 = local write "FIB HW Config"(w317) -> ()
      n160 = local write "Auto Optimzation"(w111) -> ()
      n161 = local write "3D image paused armed"(w111) -> ()
      n162 = local write "FIB emission limit warning armed"(w111) -> ()
      n163 = local write "SW error warning armed"(w111) -> ()
      n164 = local write "SEM shutter warning armed"(w111) -> ()
      n165 = local write "Focus index warning armed"(w111) -> ()
      n166 = local write "Re-engage warning armed"(w111) -> ()
      n167 = local write "FIB emission limit warning active"(w99) -> ()
      n168 = local write "SW error warning active"(w99) -> ()
      n169 = local write "SEM shutter failed active"(w99) -> ()
      n170 = local write "Focus index recovery active"(w99) -> ()
      n171 = local write "Focus index warning active"(w99) -> ()
      n172 = local write "Temperature recovery active"(w99) -> ()
      n173 = local write "Temperature warning active"(w99) -> ()
      n174 = local write "Beam dump at zero"(w99) -> ()
      n175 = local write "EHT off"(w99) -> ()
      n176 = local write "Temperature warning armed"(w99) -> ()
      n177 = local write "Auto Align"(w99) -> ()
      n178 = local write "Auto re-engage"(w99) -> ()
      n179 = local write "Off"(w99) -> ()
      n180 = local write "Spot"(w99) -> ()
      n181 = local write "Auto Stig"(w99) -> ()
      n182 = local write "FIB Profile"(w99) -> ()
      n183 = shared-variable "My Computer\\Zeiss Library.lvlib\\Milling Line Paused"(w99) -> ()  [unwired: 1 in, 1 out]
      n184 = local write "dat to csv and xml"(w99) -> ()
      n185 = local write "Send reheat start email"(w99) -> ()
      n186 = local write "Mouse down"(w99) -> ()
      n187 = local write "SEM Status"(w304) -> ()
      n188 = call-poly <vilib>:"DAQmx Create Virtual Channel.vi"("physical channels"=w100) -> ("task out"=w254:refnum<k21>, "error out"=w255:errorcluster)  [unwired: 13 in]
      n189 = local write "Mill Stop"(w99) -> ()
      n190 = local write "Stop"(w99) -> ()
      n191 = local write "ROI"(w99) -> ()
      n192 = property on="Reheat Parameters" class="Clust (strict)"("Visible"=w158) -> ()  [unwired: 2 in, 2 out]
      n193 = property on="FIB Parameters" class="Clust (strict)"("Visible"=w160) -> ()  [unwired: 2 in, 2 out]
      n194 = property on="HV Data Output" class="Clust (strict)"("Visible"=w159) -> ()  [unwired: 2 in, 2 out]
      n195 = property on="Capella HV Data Output" class="Clust (strict)"("Visible"=w101) -> ()  [unwired: 2 in, 2 out]
      n196 = Unbundle By Name(w255) -> ("status"=w253:bool)
      n197 = local write "Auto Focus"(w99) -> ()
      n198 = shared-variable "My Computer\\Zeiss Library.lvlib\\Stop"(w99) -> ()  [unwired: 1 in, 1 out]
      n199 = local write "Scan x1"(w99) -> ()
      n200 = local write "FIB time lapse"(w99) -> ()
      n201 = local write "Reheat from last"(w99) -> ()
      n202 = local read "FIB Scan Parameters"() -> (w295:T32)
      n203 = expression code="x/2"(w258) -> (w259:dbl)
      n204 = local write "Request to reheat"(w99) -> ()
      n205 = local write "Mill"(w99) -> ()
      n206 = case shown="False" w253 {
        tunnel: w254 -> [w578 _]
        frame False {
          n207 = call <vilib>:"DAQmx Clear Task.vi"("task in"=w578) -> ()  [unwired: 14 in, 1 out]
          n208 = property on="Sweep enabled" class="Bool (strict)"("DisabledEnum"=T44."Enabled" ("Disabled")) -> ()  [unwired: 2 in, 2 out]
        }
        frame True {
          n209 = local write "Sweep enabled"(FALSE ("Sweep enabled")) -> ()
          n210 = property on="Sweep enabled" class="Bool (strict)"("DisabledEnum"=T44."Disabled and Grayed Out" ("Disabled")) -> ()  [unwired: 2 in, 2 out]
        }
      }
      n211 = property on="COM port" class="VISAName"("DisabledEnum"=w257) -> ()  [unwired: 2 in, 2 out]
      n212 = local write "Re-engage cancelled"(w99) -> ()
      n213 = local write "Focus index stop trigger active"(w99) -> ()
      n214 = local read "Milling para"() -> (w291:T35)
      n215 = Bundle By Name(cluster=w291, "FIB FOV (um)"=w258, "Mill from Bottom"=FALSE, "X size (um)"=w259, "Z size (um)"=w259) -> (w290:T35)
      n216 = local read "Alert Settings"() -> (w215:T36)
      n217 = Bundle By Name(cluster=w215, "Low limit"=w214, "High limit"=w213) -> (w212:T36)
      n218 = local read "SEM Options"() -> (w284:T27)
      n219 = property on="Start FIB HV DataLog" class="Bool (strict)"("Visible"=w188) -> ()  [unwired: 2 in, 2 out]
      n220 = property on="Low limit" class="DigNum (strict)"("Caption.Text"=w224) -> ()  [unwired: 2 in, 2 out]
      n221 = property on="High limit" class="DigNum (strict)"("Caption.Text"=w223) -> ()  [unwired: 2 in, 2 out]
      n222 = property on="Faraday Cup (nA)" class="DigNum (strict)"("Caption.Text"=w221) -> ()  [unwired: 2 in, 2 out]
      n223 = property on="Faraday Cup log" class="XYGraph (strict)"("YScale.NameLbl.Text"=w220) -> ()  [unwired: 2 in, 2 out]
      n224 = property on="Config Tabs" class="TabCtl (strict)"() -> ("Pages"=w193:refnum<vi>[])  [unwired: 2 in, 2 out]
      n225 = local write "FIB"(w99) -> ()
      n226 = Bundle By Name(cluster=w295, "X size (V)"=w293, "Z size (V)"=w293) -> (w294:T32)
      n227 = local write "Mill Manual Pause"(w99) -> ()
      n228 = local write "FIB-SEM Angle"(w292) -> ()
      n229 = local read "FIB Options"() -> (w288:T33)
      n230 = property on="SEM HV Data Output" class="Clust (strict)"("Visible"=w101) -> ()  [unwired: 2 in, 2 out]
      n231 = local write "3D FIB-SEM"(w99) -> ()
      n232 = local write "Pause for reheat"(w99) -> ()
      n233 = local write "Request to stop reheat"(w99) -> ()
      n234 = property on="Extractor (kV)" class="DigNum (strict)"("Visible"=w181) -> ()  [unwired: 2 in, 2 out]
      n235 = Bundle By Name(cluster=w288, "Flip x"=w151, "Flip z"=TRUE ("data")) -> (w287:T33)
      n236 = Index Array(array=w193, index=T43."FIB Reheat" ("Config Tabs")) -> (element=w192:refnum<vi>)
      n237 = local write "Alert Settings"(w212) -> ()
      n238 = Bundle By Name(cluster=w284, "Detector A"=w282, "Detector B"=w281) -> (w283:T27)
      n239 = local read "Milling para"() -> (w302:T35)
      n240 = Bundle By Name(cluster=w302, "Auto pause"=w240, "Mill start from Last"=w240) -> (w301:T35)
      n241 = local write "Start Current DataLog"(w99) -> ()
      n242 = xnode "Match Regular Expression"("input string"=w165, "regular expression"="Merlin", "ignore case? (F)"=TRUE) -> ("offset past match"=w251:i32)  [unwired: 3 in, 4 out]
      n243 = xnode "Match Regular Expression"("input string"=w165, "regular expression"="Gemini", "ignore case? (F)"=TRUE) -> ("offset past match"=w167:i32)  [unwired: 3 in, 4 out]
      n244 = local write "Milling para"(w290) -> ()
      n245 = property class="Page"(reference=w192, "PageEnb"=w127) -> ()  [unwired: 1 in, 2 out]
      n246 = local write "FIB Imaging"(w99) -> ()
      n247 = property on="Turn FIB gun standby" class="Bool (strict)"("Visible"=w101) -> ()  [unwired: 2 in, 2 out]
      n248 = local write "FIB Options"(w287) -> ()
      n249 = Equal?(x=w251, y=-1) -> (x = y?=w164:bool)
      n250 = Equal?(x=w167, y=-1) -> (x = y?=w163:bool)
      n251 = local write "FIB Scan Parameters"(w294) -> ()
      n252 = local write "Cancel Auto re-engage"(w99) -> ()
